vi "DOE Extract Weight Data.vi"(8 "Error In":errorcluster, 10 "Weight Data":string[][](array[string]), 11 "Total Array":string[][](array[string])) -> (0 "Error Out":errorcluster, 1 "Net Weight (lbs)":dbl, 2 "Gross Weight (lbs)":dbl, 3 "Total Array Output":string[][](array[string]))   [LabVIEW 2020]
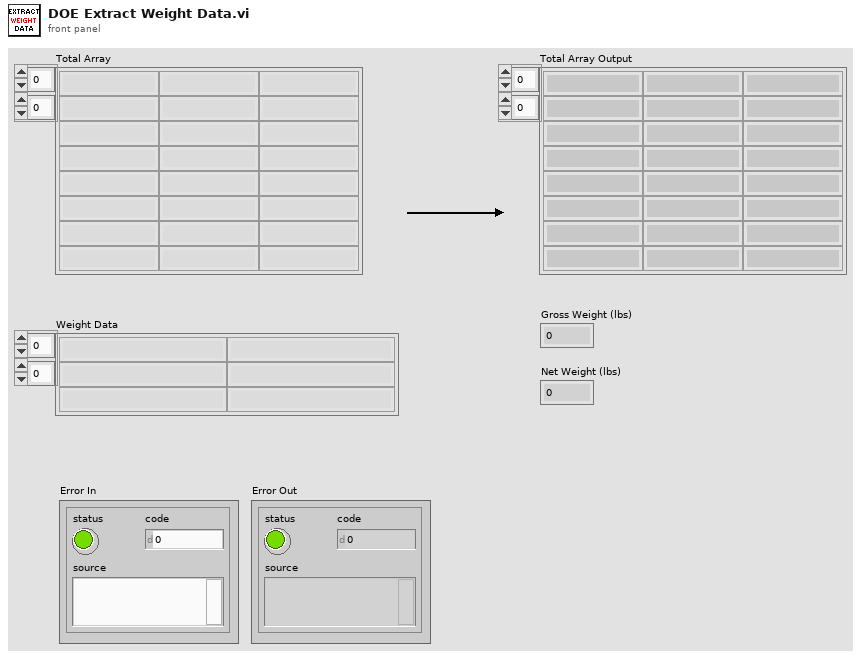
[diagram p1: front panel]
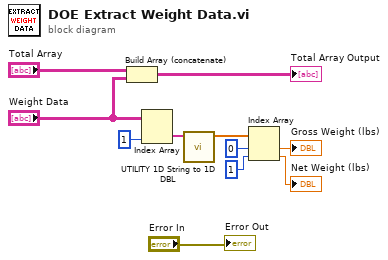
[diagram p0: block diagram]
diagram:
  n1 = Build Array (concatenate)("Total Array", "Weight Data") -> (→"Total Array Output":string[][])
  n2 = Index Array(array="Weight Data", index (col)=1 ("disabled index (col)")) -> (element=w4:string[])  [unwired: 1 in]
  n3 = call "UTILITY 1D String to 1D DBL.vi"("Save Data"=w4) -> ("DBL"=w5:dbl[])  [unwired: 10 in]
  n4 = Index Array(array=w5, index #1=0 ("index"), index #2=1 ("index")) -> (element #1=→"Gross Weight (lbs)":dbl, element #2=→"Net Weight (lbs)":dbl)
  "Error Out" <- "Error In"
